vi "Feedback_node.vi"() -> ()   [LabVIEW 2019]
panel:
  out "Factorial":i32
  in  "Input":i32
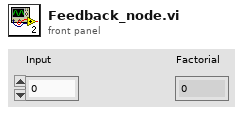
[diagram p1: front panel]
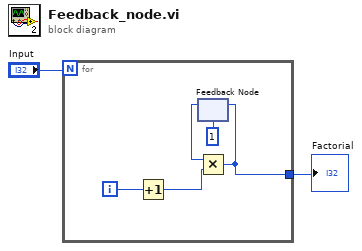
[diagram p0: block diagram]
diagram:
  n1 = for {
    N: "Input" -> [_]
    tunnel: [w3] -> w1
    i -> [w7]
    n2 = Increment(x=w7) -> (x+1=w6:i32)
    n3 = feedback #1(1) -> (w5:i32)
    n4 = Multiply(x=w5, y=w6) -> (x*y=w3:i32)
    n5 = feedback-in #1(w3) -> ()
  }
  "Factorial" <- w1
